vi "MGCC_PlannedISD_global.vi"() -> ()   [LabVIEW 2016]
panel:
  out "Grid_interface":dbl
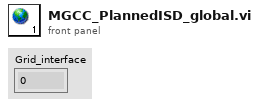
[diagram p1: front panel]
diagram:
